vi "New Component.vi"(8 "error in (no error)":errorcluster, 10 "name":string, 11 "type":T1=enum."data") -> (0 "error out":errorcluster, 3 "CycloneDX Component out":refnum<class "CycloneDX Component.lvclass">)   [LabVIEW 2017, in "LabVIEW CycloneDX SBOM.lvlib" / "CycloneDX Component.lvclass"]
uses:
  CycloneDX Component.lvclass
  C:/LabVIEW Working Directory/VIPC Software BOM/CycloneDX/CycloneDX JSON/CycloneDX JSON.lvclass
  CycloneDX JSON/CycloneDX Types.ctl
  CycloneDX JSON/CycloneDX JSON.lvclass
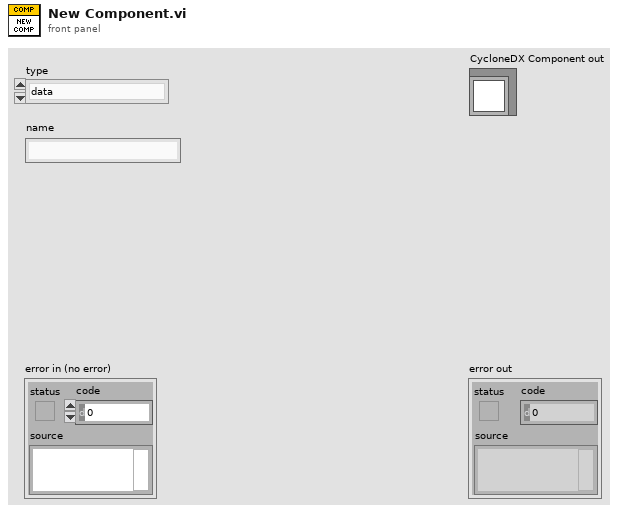
[diagram p1: front panel]
types:
  T1 = typedef "LabVIEW CycloneDX SBOM.lvlib/CycloneDX JSON.lvclass/CycloneDX Types.ctl" = enum16{"application", "framework", "library", "container", "platform", "operating-system", "device", "device-driver", "firmware", "file", "machine-learning-model", "data"}
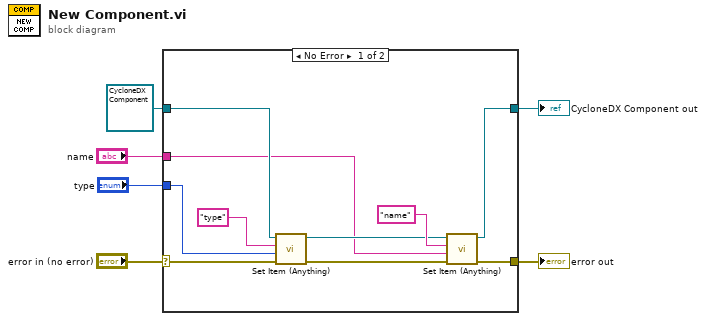
[diagram p0: block diagram]
diagram:
  n1 = case shown="No Error" "error in (no error)" {
    selector: "error in (no error)" -> [w10 w18]
    tunnel: [w11 w18] -> w5
    tunnel: [w13 w17] -> w3
    tunnel: refnum<class "CycloneDX Component.lvclass"> refnum ("CycloneDX Component in") -> [w14 w17]
    tunnel: "type" -> [w8 _]
    tunnel: "name" -> [w7 _]
    frame No Error {
      n2 = call "Set Item (Anything).vi"("error in (no error)"=w10, "Value"=w8, "Object (or Item) Path"="type", "CycloneDX SBOM in"=w14) -> ("error out"=w12:errorcluster, "CycloneDX SBOM out"=w15:refnum<class "CycloneDX Component.lvclass">)  [unwired: 6 in]
      n3 = call "Set Item (Anything).vi"("error in (no error)"=w12, "Value"=w7, "Object (or Item) Path"="name", "CycloneDX SBOM in"=w15) -> ("error out"=w11:errorcluster, "CycloneDX SBOM out"=w13:refnum<class "CycloneDX Component.lvclass">)  [unwired: 6 in]
    }
    frame Error {
    }
  }
  "error out" <- w5
  "CycloneDX Component out" <- w3
